vi "Initialize.vi"(8 "error in (no error)":errorcluster caption="错误输入（无错误）", 11 "2601B 输入":refnum<class "2601B.lvclass">) -> (0 "error out":errorcluster caption="错误输出", 3 "2601B 输出":refnum<class "2601B.lvclass">)   [LabVIEW 2020, in "2601B.lvclass"]
uses:
  2601B.lvclass
  2601B.lvclass/2601B.ctl
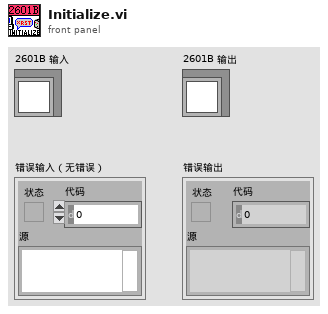
[diagram p1: front panel]
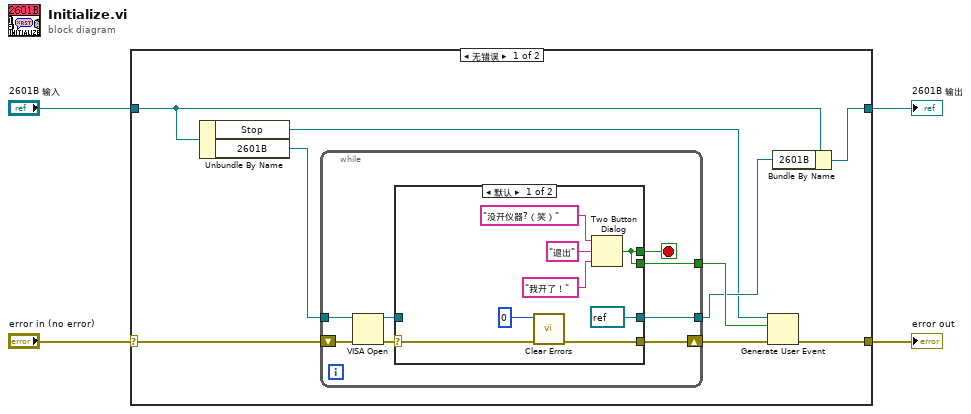
[diagram p0: block diagram]
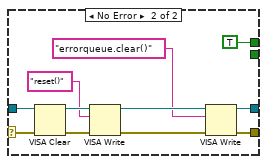
[diagram p2: hidden frame]
diagram:
  n1 = case shown="无错误" "error in (no error)" {
    selector: "error in (no error)" -> [w13 w42]
    tunnel: [w9 w42] -> w3
    tunnel: [w7 w41] -> w1
    tunnel: "2601B 输入" -> [w11 w41]
    frame No Error {
      n2 = Unbundle By Name(w11) -> ("Stop"=w5:refnum<user-event>, "2601B"=w10:refnum<visa-resource-name>)
      n3 = while {
        shift-right: [w21] -> w12
        shift-left: w13 -> [w17]
        tunnel: [w19] -> w8
        tunnel: w10 -> [w15]
        tunnel: [w14] -> w6
        stop <- w20 stop-if-true
        n4 = VISA Open(error in (no error)=w17, VISA resource name=w15) -> (VISA resource name=w18:refnum<visa-resource-name>, error out=w16:errorcluster)  [unwired: 3 in]
        n5 = case shown="默认" w16 {
          selector: w16 -> [w28 w31]
          tunnel: [w26 w34] -> w21
          tunnel: [w23 TRUE] -> w20
          tunnel: [w23 _] -> w19
          tunnel: w18 -> [_ w32]
          tunnel: [refnum<visa-resource-name> refnum ("2601B") w30] -> w14
          frame Default {
            n6 = call <vilib>:"Clear Errors.vi"("error in (no error)"=w28, "specific error code to clear (0: all)"=0) -> ("error out"=w26:errorcluster)  [unwired: 4 in, 1 out]
            n7 = Two Button Dialog(message="没开仪器?（笑）" ("消息"), 1:"我开了！" ("T按钮名称（“确定”）"), 2:"退出" ("F按钮名称（“取消”）")) -> (T button?=w23:bool)
          }
          frame No Error {
            n8 = VISA Clear(VISA resource name=w32, error in (no error)=w31) -> (VISA resource name out=w40:refnum<visa-resource-name>, error out=w39:errorcluster)
            n9 = VISA Write(VISA resource name=w40, write buffer="reset()" ("写入缓冲区"), error in (no error)=w39) -> (VISA resource name out=w36:refnum<visa-resource-name>, error out=w35:errorcluster)  [unwired: 1 out]
            n10 = VISA Write(VISA resource name=w36, write buffer="errorqueue.clear()" ("写入缓冲区"), error in (no error)=w35) -> (VISA resource name out=w30:refnum<visa-resource-name>, error out=w34:errorcluster)  [unwired: 1 out]
          }
        }
      }
      n11 = Generate User Event(user event=w5, event data cluster=w8, error in=w12) -> (error out=w9:errorcluster)  [unwired: 1 in, 1 out]
      n12 = Bundle By Name(cluster=w11, "2601B"=w6) -> (w7:refnum<class "2601B.lvclass">)
    }
    frame Error {
    }
  }
  "error out" <- w3
  "2601B 输出" <- w1
